vi "Find Command Names.vi"(10 "project root path":path, 11 "TargetItem in":refnum<vi>) -> (2 "Paths":path[](array[path]), 3 "Command Info":T2(array[cluster]))   [LabVIEW 2025]
uses:
  <vilib>/picture/picture.llb/imagedata.ctl
  <vilib>/Utility/Data Type/NI_Data Type.lvlib
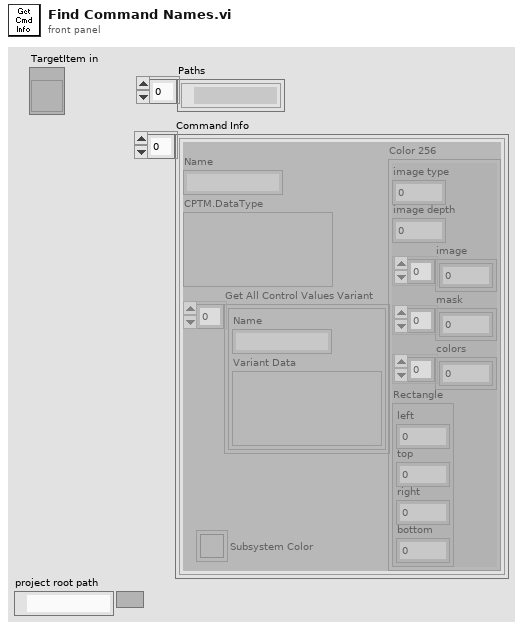
[diagram p1: front panel]
types:
  T1 = typedef "imagedata.ctl" = cluster{"image type":i32, "image depth":i32, "image":u8[], "mask":u8[], "colors":u32[], "Rectangle":cluster{"left":i16, "top":i16, "right":i16, "bottom":i16}}
  T2 = cluster{"Name":string, "CPTM.DataType":variant, "Get All Control Values Variant":cluster{"Name":string, "Variant Data":variant}[], "Color 256":T1, "Subsystem Color":u32}[]
  T3 = typedef "NI_Data Type.lvlib/Type Definition Info.ctl" = cluster{"Name":string, "Timestamp":u32}
  T4 = cluster{"Name":string, "CPTM.DataType":variant, "Get All Control Values Variant":cluster{"Name":string, "Variant Data":variant}[], "ImageData":T1, "Color Box":u32}
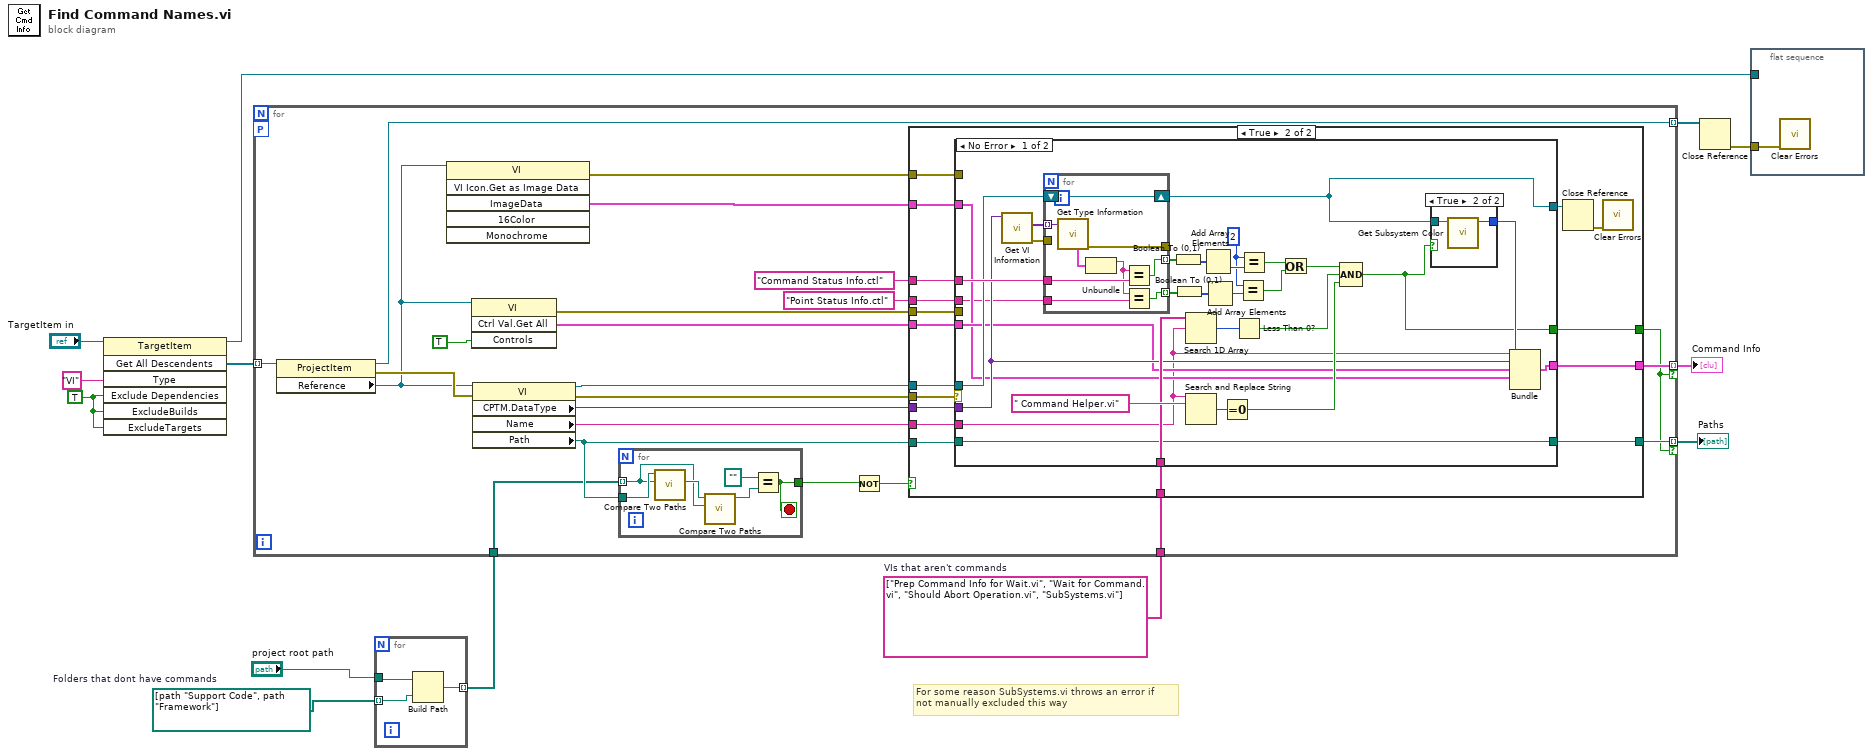
[diagram p0: block diagram]
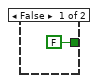
[diagram p2: hidden frame]
diagram:
  w3 = path[] [path "Support Code", path "Framework"]  # Folders that dont have commands
  w10 = TRUE ("ExcludeDependencies")
  w8 = string[] ["Prep Command Info for Wait.vi", "Wait for Command.vi", "Should Abort Operation.vi", "SubSystems.vi"]  # VIs that aren't commands
  # "For some reason SubSystems.vi throws an error if \nnot manually excluded this way"
  n1 = invoke class="TargetItem" method="Get All Descendents"(reference="TargetItem in", "Type"="VI", "Exclude Dependencies"=w10, "ExcludeBuilds"=w10, "ExcludeTargets"=w10) -> (reference out=w4:refnum<vi>, "All Descendents"=w11:refnum<vi>[])  [unwired: 2 in, 5 out]
  n2 = for {
    tunnel: w3 -> [w16] mode=indexing
    tunnel: "project root path" -> [w15]
    tunnel: [w14] -> w1 mode=indexing
    n3 = Build Path(base path=w15, name or relative path=w16) -> (appended path=w14:path)
  }
  n4 = for {
    tunnel: w11 -> [w39] mode=indexing
    tunnel: w8 -> [w37]
    tunnel: [w32] -> w12 mode=indexing if=w22
    tunnel: [w31] -> w13 mode=indexing if=w22
    tunnel: [w24] -> w5 mode=indexing
    tunnel: w1 -> [w20]
    workers-P: _ -> [_]
    n5 = property class="ProjectItem"(reference=w39) -> (reference out=w24:refnum<vi>, error out=w34:errorcluster, "Reference"=w27:refnum<vi>)  [unwired: 1 in]
    n6 = invoke class="VI" method="VI Icon.Get as Image Data"(reference=w27) -> (error out=w25:errorcluster, "ImageData"=w26:T1)  [unwired: 5 in, 4 out]
    n7 = invoke class="VI" method="Ctrl Val.Get All"(reference=w27, "Controls"=TRUE) -> (error out=w28:errorcluster, "Get All Control Values Variant"=w29:cluster{"Name":string, "Variant Data":variant}[])  [unwired: 2 in, 2 out]
    n8 = property class="VI"(reference=w27, error in=w34) -> (reference out=w23:refnum<vi>, error out=w33:errorcluster, "CPTM.DataType"=w36:variant, "Name"=w35:string, "Path"=w21:path)
    n9 = for {
      tunnel: w20 -> [w103] mode=indexing
      tunnel: w21 -> [w105]
      tunnel: [w100] -> w18
      stop <- w100 stop-if-true
      n10 = call <vilib>:"Compare Two Paths.vi"("Path 2"=w103, "Path 1"=w105) -> ("Common Path"=w104:path)  [unwired: 6 in, 3 out]
      n11 = call <vilib>:"Compare Two Paths.vi"("Path 2"=w103, "Path 1"=w104) -> ("Relative Path from 1 to 2"=w102:path)  [unwired: 6 in, 3 out]
      n12 = Equal?(x=path "", y=w102) -> (x = y?=w100:bool)
    }
    n13 = Not(x=w18) -> (.not. x?=w19:bool)
    n14 = case shown="True" w19 {
      tunnel: "Command Status Info.ctl" ("Name") -> [_ w57]
      tunnel: w37 -> [_ w56]
      tunnel: w36 -> [_ w55]
      tunnel: w35 -> [_ w54]
      tunnel: w33 -> [_ w51]
      tunnel: [_ w50] -> w32
      tunnel: [_ w49] -> w31
      tunnel: w29 -> [_ w48]
      tunnel: w28 -> [_ w47]
      tunnel: w26 -> [_ w46]
      tunnel: w25 -> [_ w45]
      tunnel: w23 -> [_ w44]
      tunnel: [FALSE w43] -> w22
      tunnel: w21 -> [_ w42]
      tunnel: "Point Status Info.ctl" -> [_ w41]
      frame False {
      }
      frame True {
        n15 = case shown="No Error" w51 {
          tunnel: w57 -> [w79 _]
          tunnel: w56 -> [w78 _]
          tunnel: w55 -> [w73 _]
          tunnel: w54 -> [w68 _]
          tunnel: [w70 w99] -> w52
          tunnel: w44 -> [w76 w99]
          tunnel: [w74 _] -> w50
          tunnel: w42 -> [w75 _]
          tunnel: [w75 _] -> w49
          tunnel: w48 -> [w72 _]
          tunnel: w47 -> [_ _]
          tunnel: w46 -> [w71 _]
          tunnel: w45 -> [_ _]
          tunnel: [w67 _] -> w43
          tunnel: w41 -> [w64 _]
          frame No Error {
            w60 = 2
            n16 = call <vilib>:"Get VI Information.vi"("variant"=w73) -> ("error out"=w82:errorcluster, "VI terminal types"=w81:variant[])  [unwired: 7 in, 2 out]
            n17 = for {
              tunnel: w79 -> [w98]
              tunnel: [w97] -> w80 mode=indexing
              tunnel: w81 -> [w95] mode=indexing
              tunnel: w82 -> [_]
              tunnel: [w94] -> _
              shift-right: [w96] -> w70
              shift-left: w76 -> [w96]
              tunnel: w64 -> [w91]
              tunnel: [w90] -> w62 mode=indexing
              n18 = call <vilib>:"Get Type Information.vi"("variant"=w95) -> ("error out"=w94:errorcluster, "type definition info"=w93:T3)  [unwired: 6 in, 3 out]
              n19 = Unbundle(w93) -> ("Name"=w92:string)  [unwired: 1 out]
              n20 = Equal?(x=w92, y=w98) -> (x = y?=w97:bool)
              n21 = Equal?(x=w92, y=w91) -> (x = y?=w90:bool)
            }
            n22 = Boolean To (0,1)(Boolean=w80) -> (0, 1=w77:i16[])
            n23 = Boolean To (0,1)(Boolean=w62) -> (0, 1=w63:i16[])
            n24 = Search 1D Array(1D array=w78, element=w68) -> (index of element=w84:i32)  [unwired: 1 in]
            n25 = Search and Replace String(input string=w68, search string=" Command Helper.vi") -> (number of replacements=w86:i32)  [unwired: 6 in, 3 out]
            n26 = Add Array Elements(numeric array=w77) -> (sum=w65:i16)
            n27 = Add Array Elements(numeric array=w63) -> (sum=w61:i16)
            n28 = Equal To 0?(x=w86) -> (x = 0?=w87:bool)
            n29 = Less Than 0?(x=w84) -> (x < 0?=w85:bool)
            n30 = Equal?(x=w60, y=w61) -> (x = y?=w59:bool)
            n31 = Equal?(x=w60, y=w65) -> (x = y?=w66:bool)
            n32 = Or(x=w66, y=w59) -> (x .or. y?=w58:bool)
            n33 = Compound Arithmetic op=AND(w58, w85, w87) -> (w67:bool)
            n34 = case shown="True" w67 {
              tunnel: w70 -> [_ w89]
              tunnel: [_ w88] -> w69
              frame False {
              }
              frame True {
                n35 = call "Get Subsystem Color.vi"("VI in"=w89) -> ("Color Box"=w88:u32)  [unwired: 10 in]
              }
            }
            n36 = Bundle("Name"=w68, "CPTM.DataType"=w73, "Get All Control Values Variant"=w72, "ImageData"=w71, "Color Box"=w69) -> (w74:T4)  [unwired: 1 in]
          }
          frame Error {
          }
        }
        n37 = Close Reference(reference=w52) -> (error out=w53:errorcluster)  [unwired: 1 in]
        n38 = call <vilib>:"Clear Errors.vi"("error in (no error)"=w53) -> ()  [unwired: 5 in, 2 out]
      }
    }
  }
  "Paths" <- w13
  "Command Info" <- w12
  n39 = Close Reference(reference=w5) -> (error out=w6:errorcluster)  [unwired: 1 in]
  n40 = flat-sequence {
    tunnel: w6 -> [w106]
    tunnel: w4 -> [_]
    frame #0 {
      n41 = call <vilib>:"Clear Errors.vi"("error in (no error)"=w106) -> ()  [unwired: 5 in, 2 out]
    }
  }
